vi "Build_Asylum_SetInWave.vi"(6 "decimation":i32, 7 "whichBank":i32, 8 "error in (no error)":errorcluster, 9 "callback":string, 10 "Wave":cluster{"channelString":string, "wave":string}, 11 "eventString":string) -> (0 "error out":errorcluster, 3 "Command":string)   [LabVIEW 2019]
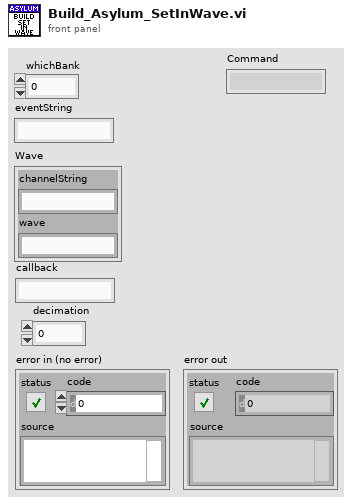
[diagram p1: front panel]
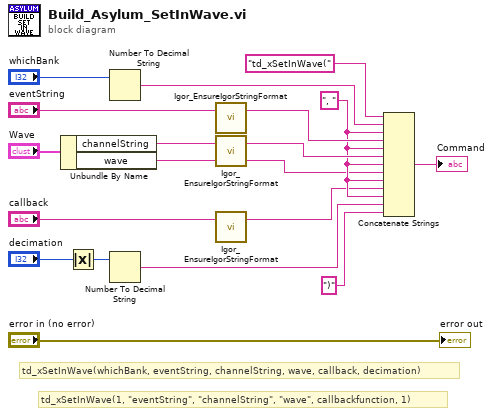
[diagram p0: block diagram]
diagram:
  w8 = ", "
  # "td_xSetInWave(1, \"eventString\", \"channelString\", \"wave\", callbackfunction, 1)"
  # "td_xSetInWave(whichBank, eventString, channelString, wave, callback, decimation)"
  n1 = Unbundle By Name("Wave") -> ("channelString"=w15:string, "wave"=w1:string)
  n2 = Absolute Value(x="decimation") -> (abs(x)=w13:i32)
  n3 = Number To Decimal String(number="whichBank") -> (decimal integer string=w11:string)  [unwired: 1 in]
  n4 = Number To Decimal String(number=w13) -> (decimal integer string=w7:string)  [unwired: 1 in]
  n5 = call <userlib>:"Igor_EnsureIgorStringFormat.vi"("Value"="eventString") -> ("Value"=w10:string)  [unwired: 2 in]
  n6 = call <userlib>:"Igor_EnsureIgorStringFormat.vi"("Value"=w15) -> ("Value"=w9:string)  [unwired: 2 in]
  n7 = call <userlib>:"Igor_EnsureIgorStringFormat.vi"("Value"="callback") -> ("Value"=w3:string)  [unwired: 2 in]
  n8 = Concatenate Strings("td_xSetInWave(" ("string"), w11, w8, w10, w8, w9, w8, w1, w8, w3, w8, w7, ")" ("string")) -> (→"Command":string)
  "error out" <- "error in (no error)"
